vi "Remove - Update Poly.vi"(7 "Poly Ref Map":T3, 8 "error in (no error)":errorcluster, 11 "Poly Set Map in":T1) -> (0 "error out":errorcluster, 3 "Poly Set Map out":T1)   [LabVIEW 2020]
uses:
  _td_cluster_InstanceInfo.ctl
  _td_map_PolyInstanceInfo.ctl
  _td_map_PolyRef.ctl
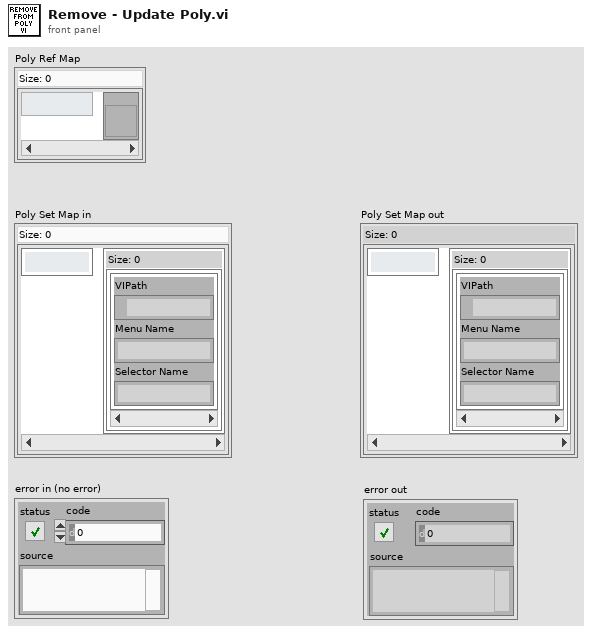
[diagram p1: front panel]
types:
  T1 = typedef "_td_map_PolyInstanceInfo.ctl" = map{string, set{T2}}
  T2 = typedef "_td_cluster_InstanceInfo.ctl" = cluster{"VIPath":path, "Menu Name":string, "Selector Name":string}
  T3 = typedef "_td_map_PolyRef.ctl" = map{string, refnum<vi>}
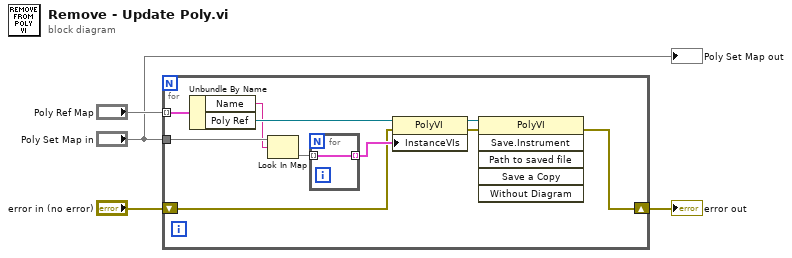
[diagram p0: block diagram]
diagram:
  n1 = for {
    tunnel: "Poly Ref Map" -> [w14] mode=indexing
    tunnel: "Poly Set Map in" -> [w12]
    shift-right: [w5] -> w2
    shift-left: "error in (no error)" -> [w7]
    n2 = Unbundle By Name(w14) -> ("Name"=w11:string, "Poly Ref"=w13:refnum<vi>)
    n3 = Look In Map(map=w12, key=w11) -> (value=w10:set{T2})  [unwired: 1 in, 1 out]
    n4 = for {
      tunnel: w10 -> [w15] mode=indexing
      tunnel: [w15] -> w9 mode=indexing
    }
    n5 = property class="PolyVI"(reference=w13, error in=w7, "InstanceVIs"=w9) -> (reference out=w8:refnum<vi>, error out=w6:errorcluster)
    n6 = invoke class="PolyVI" method="Save.Instrument"(reference=w8, error in=w6) -> (error out=w5:errorcluster)  [unwired: 4 in, 5 out]
  }
  "error out" <- w2
  "Poly Set Map out" <- "Poly Set Map in"
